vi "Wiimote Decrypt Extension Data.vi"(1 "Encrypted Data in":u8[](array[numeric]) format="%02x") -> (0 "Decrypted Data out":u8[](array[numeric]) format="%02x")   [LabVIEW 2012, in "Wiimote.lvlib"]
uses:
  Wiimote.lvlib
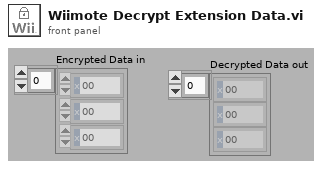
[diagram p1: front panel]
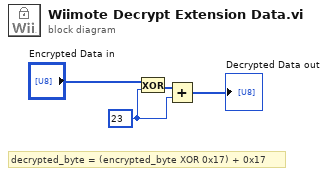
[diagram p0: block diagram]
diagram:
  w3 = u8 23 ("index")
  # "decrypted_byte = (encrypted_byte XOR 0x17) + 0x17"
  n1 = Exclusive Or(1:w3, 2:"Encrypted Data in") -> (0:w4:u8[])
  n2 = Add(x=w4, y=w3) -> (x+y=→"Decrypted Data out":u8[])
